vi "SERIAL_ValidateTermination.vi"(2 "Expected Packet Length":i32, 3 "Content":string) -> (0 "Termination Offset":i32, 1 "Valid?":bool)   [LabVIEW 2014, in "navX Library v1 (deprecated).lvlib"]
uses:
  navX Library v1 (deprecated).lvlib
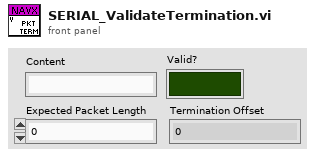
[diagram p1: front panel]
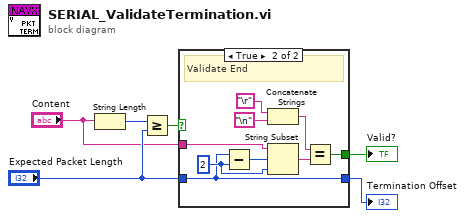
[diagram p0: block diagram]
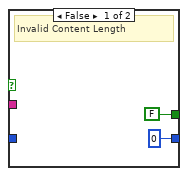
[diagram p2: hidden frame]
diagram:
  n1 = String Length(string="Content") -> (length=w6:i32)
  n2 = Greater Or Equal?(x=w6, y="Expected Packet Length") -> (x >= y?=w4:bool)
  n3 = case shown="True" w4 {
    tunnel: "Expected Packet Length" -> [_ w9]
    tunnel: "Content" -> [_ w14]
    tunnel: [FALSE w11] -> w2
    tunnel: [0 ("Expected Packet Length") w9] -> w1
    frame False {
      # "Invalid Content Length"
    }
    frame True {
      w13 = 2 ("length (rest)")
      # "Validate End"
      n4 = Subtract(x=w9, y=w13) -> (x-y=w10:i32)
      n5 = Concatenate Strings("\r", "\n") -> (w15:string)
      n6 = String Subset(string=w14, offset (0)=w10, length (rest)=w13) -> (substring=w12:string)
      n7 = Equal?(x=w15, y=w12) -> (x = y?=w11:bool)
    }
  }
  "Valid?" <- w2
  "Termination Offset" <- w1
